vi "系统设置.vi"   [LabVIEW 2016]
uses:
  <vilib>/Utility/miscctls.llb/LVPointTypeDef.ctl
  <vilib>/Utility/config.llb/NI_LVConfig.lvlib
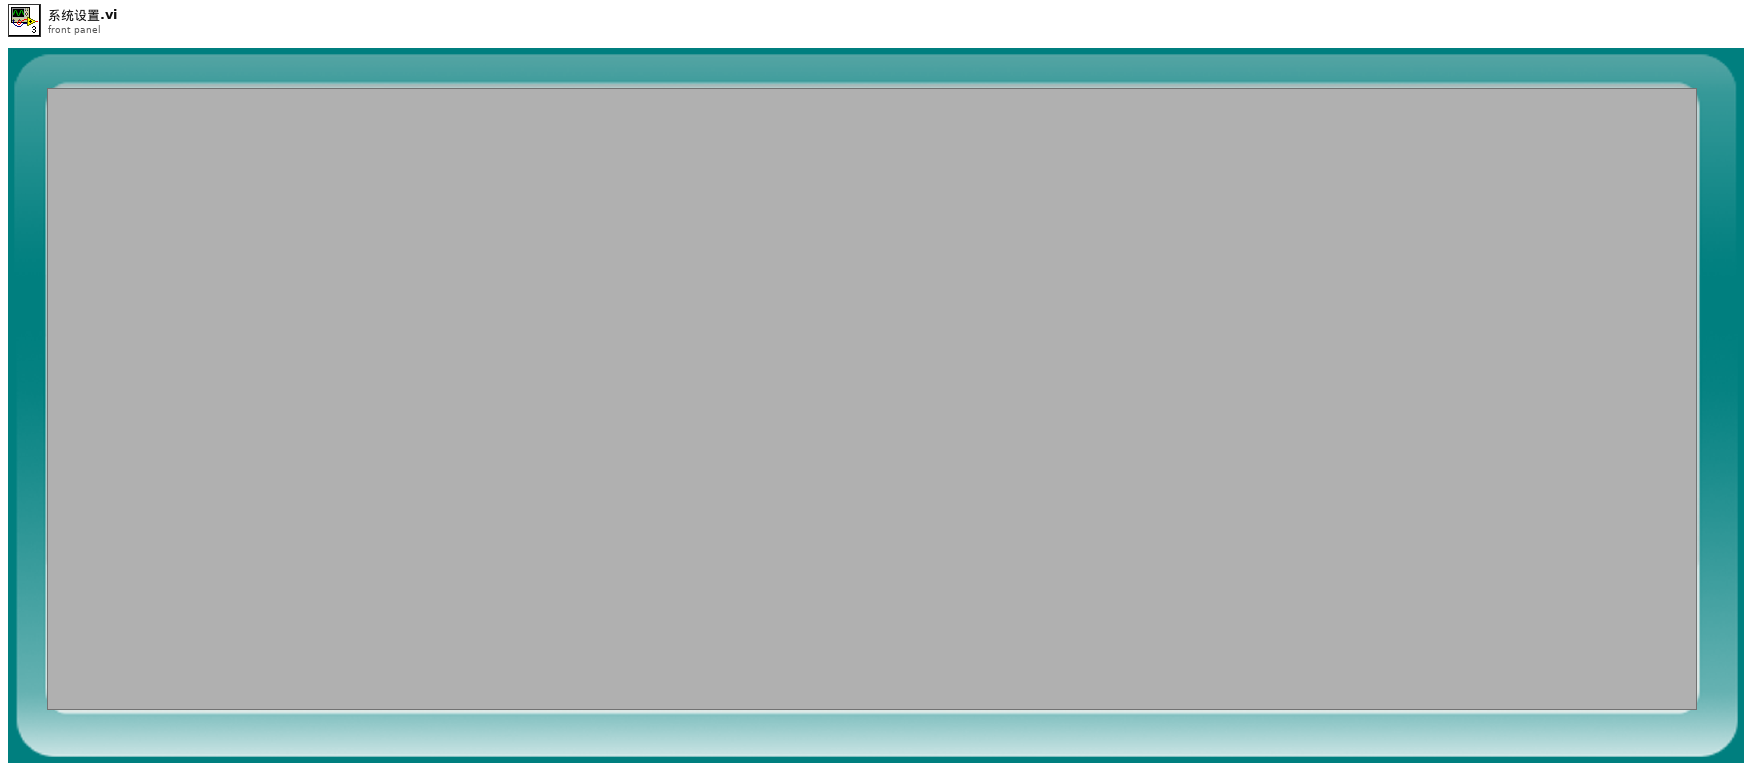
[diagram p1: front panel]
types:
  T1 = typedef "LVPointTypeDef.ctl" = cluster{"Horizontal":i16, "Vertical":i16}
  T2 = typedef "NI_LVConfig.lvlib/Config Data RefNum.ctl" = refnum<k1>
  T3 = enum32{"Bad", "Idle", "Run top level", "Running"}
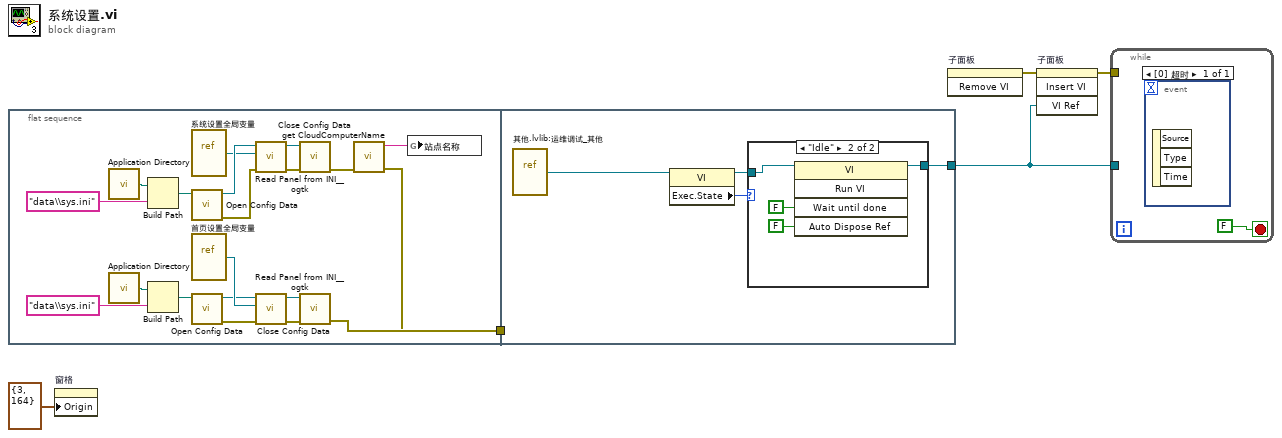
[diagram p0: block diagram]
diagram:
  n1 = flat-sequence {
    tunnel: [w10] -> w5
    tunnel: [w7] -> w4
    tunnel: [w30] -> w2
    tunnel: w5 -> [_]
    tunnel: w4 -> [_]
    frame #0 {
      n2 = call <vilib>:"Application Directory.vi"() -> ("Application Directory"=w18:path)
      n3 = call <vilib>:"Application Directory.vi"() -> ("Application Directory"=w19:path)
      n4 = Build Path(base path=w18, name or relative path="data\\sys.ini" ("名称或相对路径")) -> (appended path=w16:path)
      n5 = Build Path(base path=w19, name or relative path="data\\sys.ini" ("名称或相对路径")) -> (appended path=w21:path)
      n6 = vi-ref "系统设置全局变量.vi"() -> (w14:refnum<vi>)
      n7 = call <vilib>:"Open Config Data.vi"("configuration file path"=w16) -> ("error out"=w12:errorcluster, "refnum"=w15:T2)  [unwired: 8 in, 1 out]
      n8 = vi-ref "首页设置全局变量.vi"() -> (w23:refnum<vi>)
      n9 = call <vilib>:"Open Config Data.vi"("configuration file path"=w21) -> ("error out"=w25:errorcluster, "refnum"=w22:T2)  [unwired: 8 in, 1 out]
      n10 = call <userlib>:"Read Panel from INI__ogtk.vi"("error in (no error)"=w12, "VI ref"=w14, "refnum"=w15) -> ("error out"=w11:errorcluster, "refnum out"=w13:T2)  [unwired: 7 in]
      n11 = call <userlib>:"Read Panel from INI__ogtk.vi"("error in (no error)"=w25, "VI ref"=w23, "refnum"=w22) -> ("error out"=w26:errorcluster, "refnum out"=w24:T2)  [unwired: 7 in]
      n12 = call <vilib>:"Close Config Data.vi"("error in (no error)"=w11, "refnum"=w13) -> ("error out"=w8:errorcluster)  [unwired: 8 in, 1 out]
      n13 = call <vilib>:"Close Config Data.vi"("error in (no error)"=w26, "refnum"=w24) -> ("error out"=w10:errorcluster)  [unwired: 8 in, 1 out]
      n14 = call "get CloudComputerName.vi"("error in (no error)"=w8) -> ("error out"=w7:errorcluster, "String/Binary data"=w9:string)  [unwired: 9 in]
      n15 = global write "系统设置全局变量.vi" "站点名称"(w9) -> ()
    }
    frame #1 {
      n16 = vi-ref "其他.lvlib:运维调试_其他.vi"() -> (w27:refnum<vi>)
      n17 = property class="VI"(reference=w27) -> (reference out=w28:refnum<vi>, "Exec.State"=w29:T3)  [unwired: 1 in, 1 out]
      n18 = case shown="\"Idle\"" w29 {
        tunnel: w28 -> [w31 w33]
        tunnel: [w31 w32] -> w30
        frame "Bad", Default {
        }
        frame "Idle" {
          n19 = invoke class="VI" method="Run VI"(reference=w33, "Wait until done"=FALSE ("结束前等待"), "Auto Dispose Ref"=FALSE ("自动销毁引用")) -> (reference out=w32:refnum<vi>)  [unwired: 2 in, 4 out]
        }
      }
    }
  }
  n20 = property on="窗格" class="Pane"("Origin"=T1 {"Horizontal"=3, "Vertical"=164} ("原点")) -> ()  [unwired: 2 in, 2 out]
  n21 = invoke on="子面板" class="SubPnl" method="Remove VI"() -> (error out=w3:errorcluster)  [unwired: 3 in, 2 out]
  n22 = invoke on="子面板" class="SubPnl" method="Insert VI"(error in=w3, "VI Ref"=w2) -> (error out=w1:errorcluster)  [unwired: 2 in, 3 out]
  n23 = while {
    tunnel: w2 -> [_]
    tunnel: w1 -> [_]
    stop <- FALSE stop-if-true
    n24 = event shown="[0] 超时" {
      selector: _ -> [_]
      dyn-events: _ -> [_]
      timeout: _ -> [_]
      event Timeout {
        n25 = event-data() -> ()  [unwired: 1 in, 3 out]
      }
    }
  }
